vi "fgv_limits.vi"(7 "cmd":T2, 11 "limits":T1) -> (3 "limits 2":T1)   [LabVIEW 2019]
uses:
  _ctrl/rw.ctl
  limits.ctl
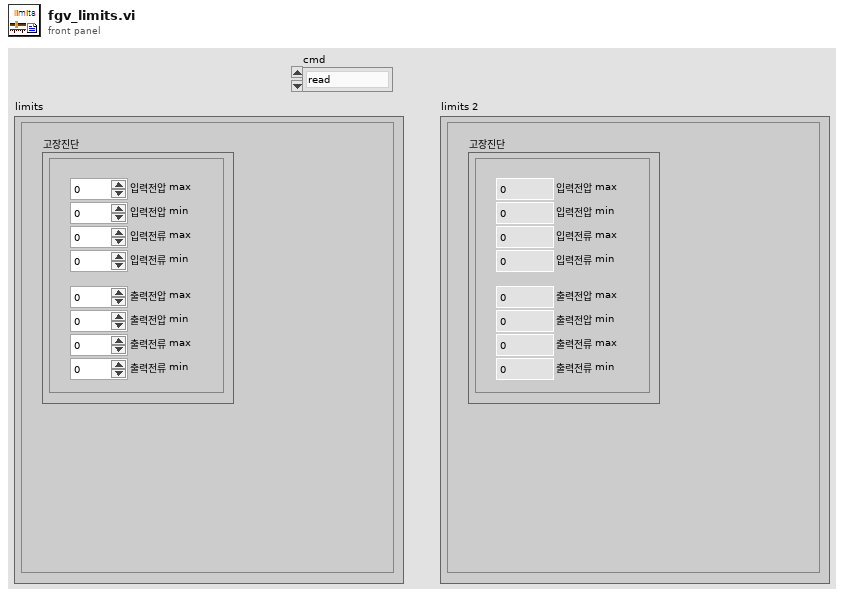
[diagram p1: front panel]
types:
  T1 = typedef "limits.ctl" = cluster{"고장진단":cluster{"입력전압 max":dbl, "입력전류 max":dbl, "출력전압 max":dbl, "출력전류 max":dbl, "입력전압 min":dbl, "입력전류 min":dbl, "출력전압 min":dbl, "출력전류 min":dbl}}
  T2 = typedef "rw.ctl" = enum16{"read", "write"}
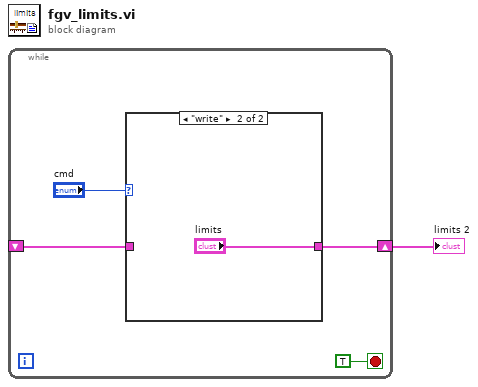
[diagram p0: block diagram]
diagram:
  n1 = while {
    shift-right: [w3] -> w1
    shift-left: _ -> [w2]
    stop <- TRUE stop-if-true
    n2 = case shown="\"write\"" "cmd" {
      tunnel: [w6 "limits"] -> w3
      tunnel: w2 -> [w6 _]
      frame "read", Default {
      }
      frame "write" {
      }
    }
  }
  "limits 2" <- w1
